vi "Module Connect.vi"(10 "Panel Info In":T2(c390), 11 "Panel Name":string[](array[string])) -> (2 "Panel Info Out":T2(c390), 3 "OK?":bool)   [LabVIEW 2020]
panel:
  in  "Mudules":T1(array[cluster]) {"Panel Name" items=["CVM数据显示", "I_V曲线", "报警日志", "参数设置", "单体电压数据源", "费思电子负载", "负载控制", "负载曲线", "控制面板", "灵活控制面板", "流程图", "数据监控", "西门子PLC", "系统数据源", "相对湿度"]}
  in  "OK":bool
  in  "Cancel":bool
  # "标签"
  # "名称"
  # "面板"
  # "使用"
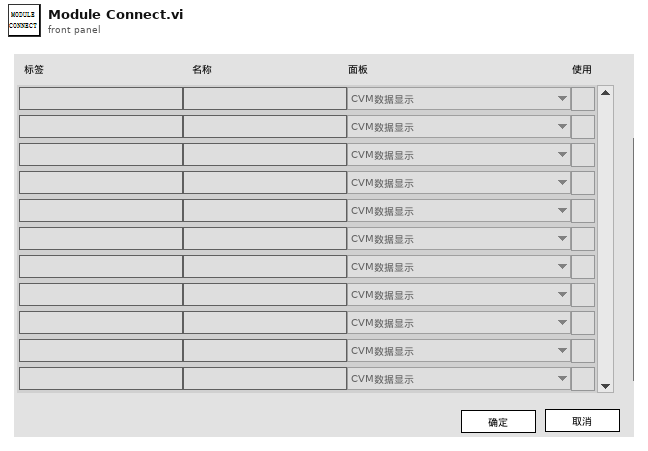
[diagram p1: front panel]
types:
  T1 = cluster{"Lable":string, "Name":string, "Panel Name":u16, "Enable":bool}[]
  T2 = map{string, cluster{"Lable":string, "Name":string, "Panel":string, "Use":string}}
  T3 = cluster{"OK?":bool, "Panel Name":string[], "Panel Info":map{string, cluster{"Lable":string, "Name":string, "Panel":string, "Use":string}}}
  T4 = cluster{"Lable":string, "Name":string, "Panel Name":u16, "Enable":bool}
  T5 = cluster{"Lable":string, "Name":string, "Panel":string, "Use":string}
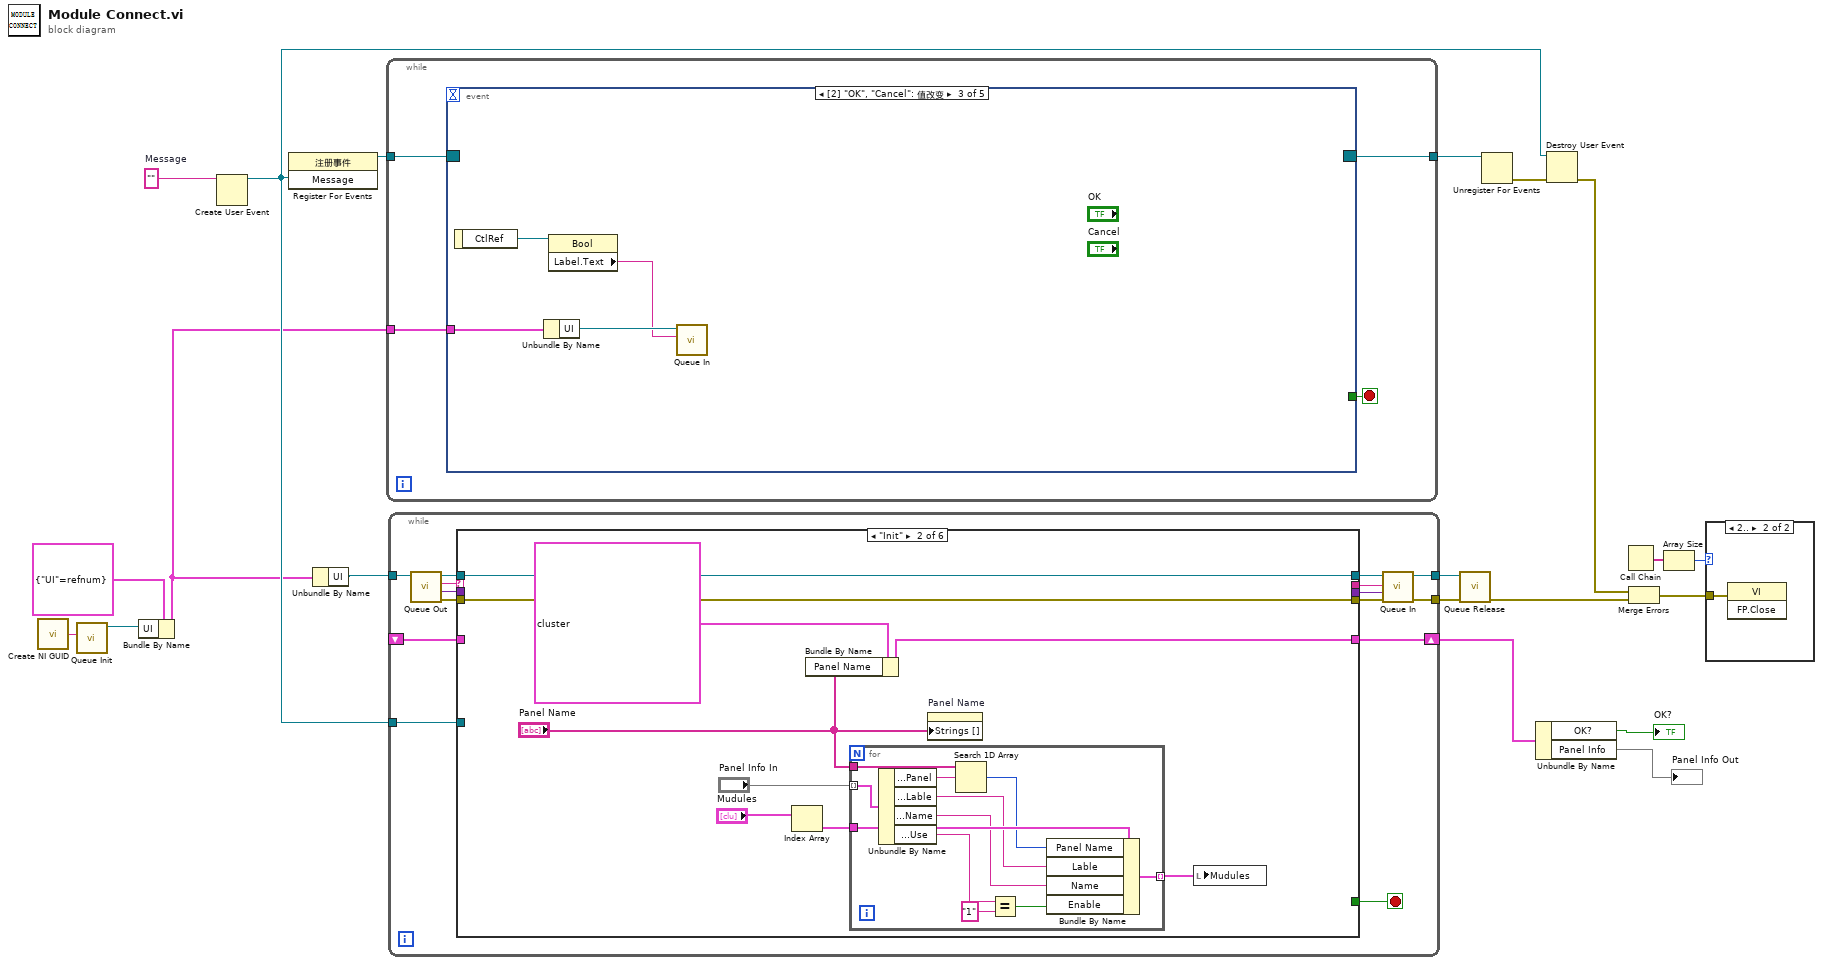
[diagram p0: block diagram]
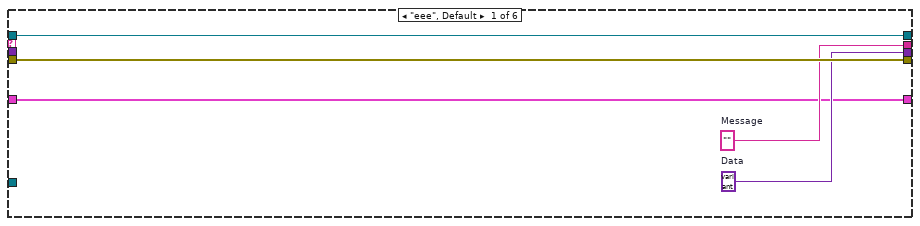
[diagram p3: hidden frame]
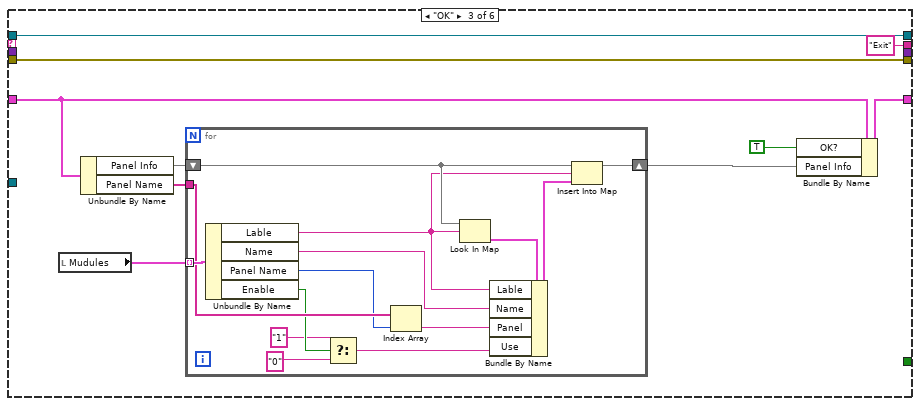
[diagram p4: hidden frame]
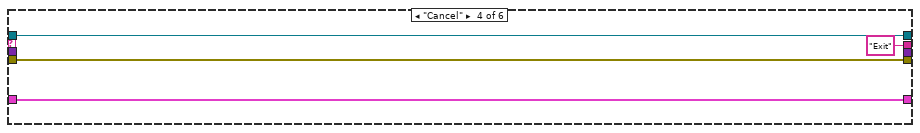
[diagram p5: hidden frame]
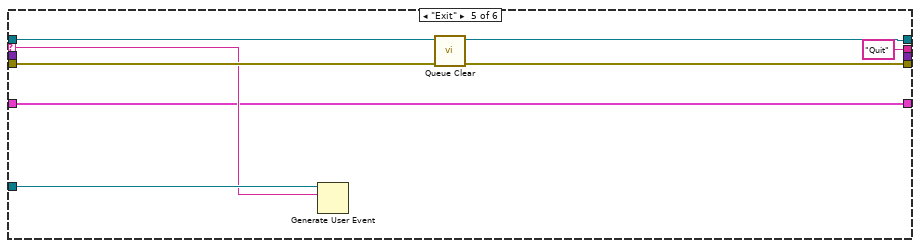
[diagram p6: hidden frame]
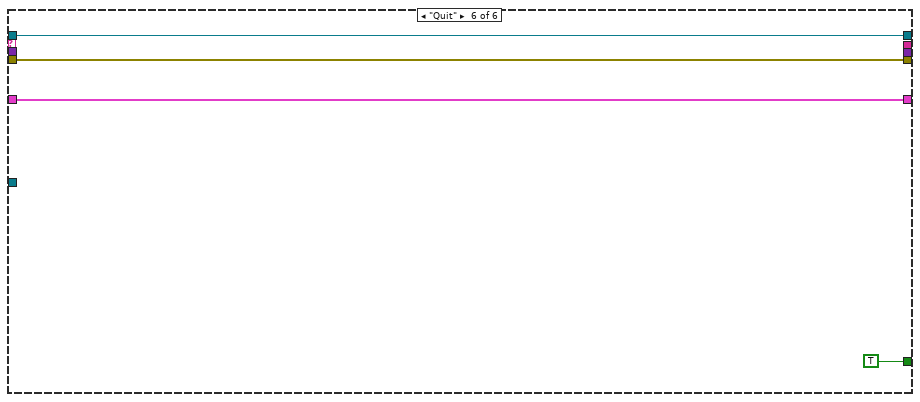
[diagram p7: hidden frame]
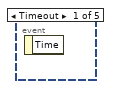
[diagram p8: hidden frame]
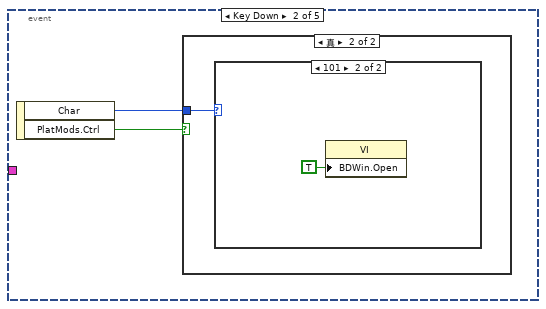
[diagram p9: hidden frame]
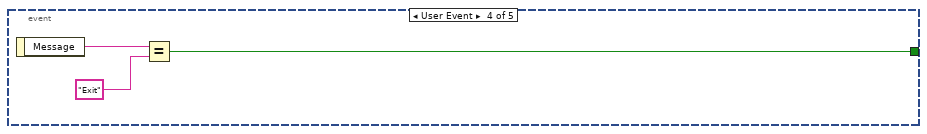
[diagram p12: hidden frame]
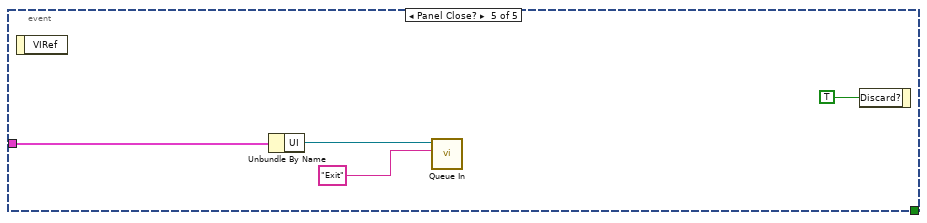
[diagram p13: hidden frame]
diagram:
  w8 = ""  # Message
  n1 = call <vilib>:"Create NI GUID.vi"() -> ("NI GUID"=w6:string)
  n2 = call "Queue Init.vi"("Queue Name"=w6) -> ("Queue Out"=w4:refnum<queue>)  [unwired: 8 in, 2 out]
  n3 = Bundle By Name(cluster=cluster{"UI":refnum<queue>} {"UI"=refnum} ("Queue Ref Out"), "UI"=w4) -> (w5:cluster{"UI":refnum<queue>})
  n4 = Create User Event(user event datatype=w8) -> (user event=w12:refnum<user-event>)  [unwired: 1 in, 1 out]
  n5 = register-events(w12) -> (reference out=w9:refnum<event-registration>)  [unwired: 2 in, 1 out]
  n6 = Unbundle By Name(w5) -> ("UI"=w15:refnum<queue>)
  n7 = while {
    tunnel: w9 -> [w24]
    tunnel: [w22] -> w10
    tunnel: w5 -> [w21]
    stop <- w23 stop-if-true
    n8 = event shown="[2] \"OK\", \"Cancel\": 值改变" {
      selector: w24 -> [_ _ _ _ _]
      dyn-events: [_ _ _ _ _] -> w22
      timeout: _ -> [_ _ _ _ _]
      tunnel: [_ _ _ w33 _] -> w23
      tunnel: w21 -> [_ _ w31 _ w38]
      event Timeout {
        n9 = event-data() -> ()  [unwired: 1 in, 1 out]
      }
      event Key Down {
        n10 = event-data() -> ("Char"=w26:i16, "PlatMods.Ctrl"=w25:bool)  [unwired: 1 in]
        n11 = case shown="真" w25 {
          tunnel: w26 -> [_ w27]
          frame False {
          }
          frame True {
            n12 = case shown="101" w27 {
              frame 0, Default {
              }
              frame 101 {
                n13 = property class="VI"("BDWin.Open"=TRUE ("程序框图窗口:打开")) -> ()  [unwired: 2 in, 2 out]
              }
            }
          }
        }
      }
      event "OK", "Cancel": Value Change {
        n14 = event-data() -> ("CtlRef"=w32:refnum<vi>)  [unwired: 1 in]
        n15 = Unbundle By Name(w31) -> ("UI"=w30:refnum<queue>)
        n16 = property class="Bool"(reference=w32) -> ("Label.Text"=w29:string)  [unwired: 1 in, 2 out]
        n17 = call "Queue In.vi"("Message"=w29, "Queue In"=w30) -> ()  [unwired: 8 in, 2 out]
      }
      event User Event {
        n18 = event-data() -> ("Message"=w35:string)  [unwired: 1 in]
        n19 = Equal?(x=w35, y="Exit") -> (x = y?=w33:bool)
      }
      event Panel Close? {
        n20 = event-data() -> ()  [unwired: 1 in, 1 out]
        n21 = Unbundle By Name(w38) -> ("UI"=w37:refnum<queue>)
        n22 = call "Queue In.vi"("Message"="Exit", "Queue In"=w37) -> ()  [unwired: 8 in, 2 out]
        n23 = event-data("Discard?"=TRUE ("放弃？")) -> ()  [unwired: 1 in, 1 out]
      }
    }
  }
  n24 = while {
    tunnel: w15 -> [w49]
    tunnel: [w46] -> w13
    tunnel: [w45] -> w14
    tunnel: w12 -> [w53]
    shift-right: [w41] -> w3
    shift-left: _ -> [w40]
    stop <- w54 stop-if-true
    n25 = call "Queue Out.vi"("Queue In"=w49) -> ("error out"=w52:errorcluster, "Data"=w50:variant, "Message"=w51:string, "Queue Out"=w48:refnum<queue>)  [unwired: 6 in, 1 out]
    n26 = case shown="\"Init\"" w51 {
      selector: w51 -> [_ _ _ _ w109 _]
      tunnel: w48 -> [w59 w68 w89 w107 w113 w118]
      tunnel: w52 -> [w58 w67 w88 w106 w111 w119]
      tunnel: [w59 w68 w89 w107 w112 w118] -> w47
      tunnel: [w58 w67 w88 w106 w110 w119] -> w44
      tunnel: [w57 _ "Exit" ("Message") "Exit" ("Message") "Quit" _] -> w43
      tunnel: [_ _ _ _ _ TRUE] -> w54
      tunnel: w53 -> [_ _ _ _ w115 _]
      tunnel: [w56 _ _ _ _ _] -> w42
      tunnel: w50 -> [_ _ _ _ _ _]
      tunnel: [w55 w65 w87 w105 w108 w116] -> w41
      tunnel: w40 -> [w55 _ w83 w105 w108 w116]
      frame "eee", Default {
        w56 = variant  # Data
        w57 = ""  # Message
      }
      frame "Init" {
        n27 = Index Array(array="Mudules") -> (element=w61:T4)  [unwired: 1 in]
        n28 = Bundle By Name(cluster=T3 {"OK?"=FALSE, "Panel Name"=[], "Panel Info"={}}, "Panel Name"="Panel Name") -> (w65:T3)
        n29 = for {
          tunnel: "Panel Info In" -> [w79] mode=indexing
          tunnel: "Panel Name" -> [w78]
          tunnel: w61 -> [w76]
          tunnel: [w69] -> w60 mode=indexing
          n30 = Unbundle By Name(w79) -> ("Panel Info.Panel"=w77:string, "Panel Info.Lable"=w74:string, "Panel Info.Name"=w73:string, "Panel Info.Use"=w72:string)
          n31 = Search 1D Array(1D array=w78, element=w77) -> (index of element=w75:i32)  [unwired: 1 in]
          n32 = Equal?(x=w72, y="1") -> (x = y?=w70:bool)
          n33 = Bundle By Name(cluster=w76, "Panel Name"=w75, "Lable"=w74, "Name"=w73, "Enable"=w70) -> (w69:T4)
        }
        n34 = property on="Panel Name" class="Ring (严格)"("Strings []"="Panel Name") -> ()  [unwired: 2 in, 2 out]
        n35 = local write "Mudules"(w60) -> ()
      }
      frame "OK" {
        n36 = local read "Mudules"() -> (w84:T1)
        n37 = Unbundle By Name(w83) -> ("Panel Info"=w82:T2, "Panel Name"=w81:string[])
        n38 = for {
          tunnel: w84 -> [w103] mode=indexing
          shift-right: [w100] -> w80
          shift-left: w82 -> [w101]
          tunnel: w81 -> [w96]
          n39 = Unbundle By Name(w103) -> ("Lable"=w98:string, "Name"=w97:string, "Panel Name"=w95:u16, "Enable"=w93:bool)
          n40 = Select(t="1", s=w93, f="0") -> (s? t:f=w90:string)
          n41 = Index Array(array=w96, index=w95) -> (element=w94:string)
          n42 = Look In Map(map=w101, key=w98) -> (value=w102:T5)  [unwired: 1 in, 1 out]
          n43 = Bundle By Name(cluster=w102, "Lable"=w98, "Name"=w97, "Panel"=w94, "Use"=w90) -> (w99:T5)
          n44 = Insert Into Map(map in=w101, key=w98, value=w99) -> (map out=w100:T2)  [unwired: 2 out]
        }
        n45 = Bundle By Name(cluster=w83, "OK?"=TRUE, "Panel Info"=w80) -> (w87:T3)
      }
      frame "Cancel" {
      }
      frame "Exit" {
        n46 = Generate User Event(user event=w115, event data cluster=w109) -> ()  [unwired: 2 in, 2 out]
        n47 = call "Queue Clear.vi"("error in (no error)"=w111, "Queue In"=w113) -> ("error out"=w110:errorcluster, "Queue Out"=w112:refnum<queue>)  [unwired: 8 in]
      }
      frame "Quit" {
      }
    }
    n48 = call "Queue In.vi"("error in (no error)"=w44, "Data"=w42, "Message"=w43, "Queue In"=w47) -> ("error out"=w45:errorcluster, "Queue Out"=w46:refnum<queue>)  [unwired: 6 in]
  }
  n49 = call "Queue Release.vi"("error in (no error)"=w14, "Queue In"=w13) -> ("error out"=w17:errorcluster)  [unwired: 9 in]
  n50 = Unregister For Events(event registration refnum=w10) -> (error out=w11:errorcluster)  [unwired: 1 in]
  n51 = Unbundle By Name(w3) -> ("OK?"=→"OK?":bool, "Panel Info"=→"Panel Info Out":T2)
  n52 = Destroy User Event(user event=w12, error in=w11) -> (error out=w16:errorcluster)
  n53 = Call Chain() -> (call chain=w19:string[])
  n54 = Merge Errors(w16, w17) -> (w18:errorcluster)
  n55 = Array Size(array=w19) -> (size(s)=w20:i32)
  n56 = case shown="2.." w20 {
    tunnel: w18 -> [_ w120]
    frame 0, Default {
    }
    frame 2.. {
      n57 = invoke class="VI" method="FP.Close"(error in=w120) -> ()  [unwired: 2 in, 3 out]
    }
  }
